vi "Add to Tree.vi"(8 "error in (no error)":errorcluster, 9 "Parent Tag":string, 10 "Tree Manager in":refnum<class "Tree Manager.lvclass">, 11 "Attribute in":refnum<class "Attribute.lvclass">) -> (0 "error out":errorcluster, 2 "Tree Manager out":refnum<class "Tree Manager.lvclass">, 3 "Attribute out":refnum<class "Attribute.lvclass">)   [LabVIEW 2023, in "VILab.lvlib" / "Attribute.lvclass"]
uses:
  Attribute.lvclass
  Tree Manager.lvclass
  Data Item.lvclass
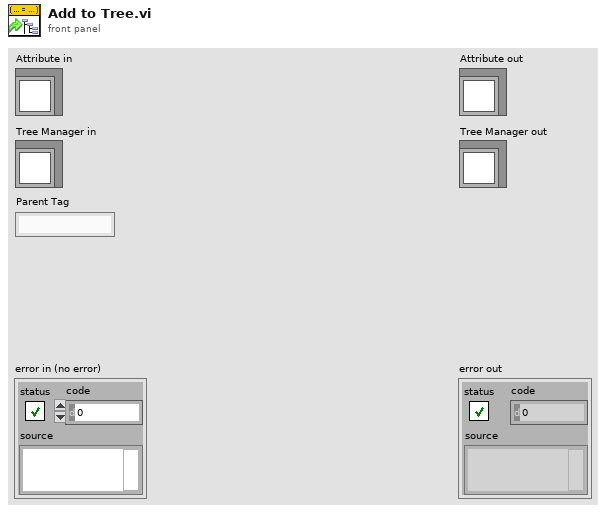
[diagram p1: front panel]
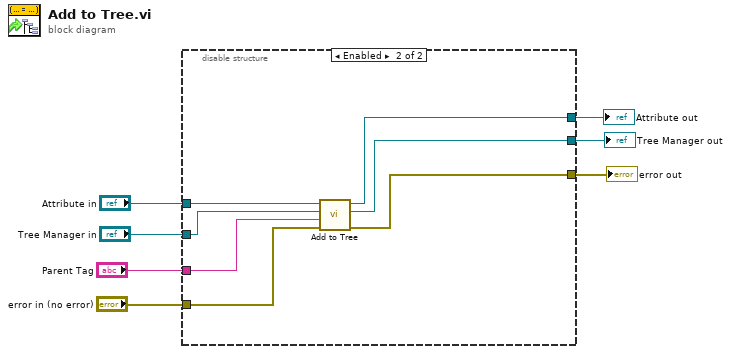
[diagram p0: block diagram]
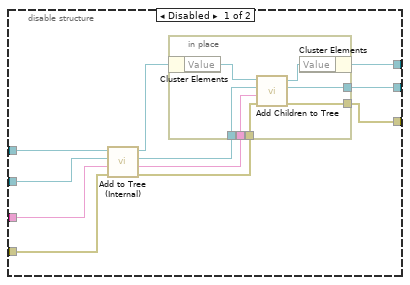
[diagram p2: hidden frame]
diagram:
  n1 = disable-structure shown="Enabled" {
    disable-tunnel: "Parent Tag" -> [w18 w30]
    disable-tunnel: "Tree Manager in" -> [w17 w31]
    disable-tunnel: "error in (no error)" -> [w16 w29]
    disable-tunnel: "Attribute in" -> [w15 w32]
    disable-tunnel: [w10 w28] -> w3
    disable-tunnel: [w9 w27] -> w2
    disable-tunnel: [w8 w26] -> w1
    frame Disabled {
      n2 = call "Add to Tree (Internal).vi"("error in (no error)"=w16, "Parent Tag"=w18, "Tree Manager in"=w17, "Data Item in"=w15) -> ("error out"=w13:errorcluster, "New Tag"=w11:string, "Tree Manager out"=w12:refnum<class "Tree Manager.lvclass">, "Data Item out"=w14:refnum<class "Attribute.lvclass">)  [unwired: 4 in]
      n3 = in-place {
        in-place-border: w13 -> [w23]
        in-place-border: w12 -> [w22]
        in-place-border: w11 -> [w21]
        in-place-border: [w20] -> w9
        in-place-border: [w19] -> w8
        n4 = in-place-cluster #1(w14) -> ("Value"=w25:refnum<class "Data Item.lvclass">)
        n5 = call "Add Children to Tree.vi"("error in (no error)"=w23, "Parent Tag"=w21, "Tree Manager in"=w22, "Data Item in"=w25) -> ("error out"=w19:errorcluster, "Tree Manager out"=w20:refnum<class "Tree Manager.lvclass">, "Data Item out"=w24:refnum<class "Data Item.lvclass">)  [unwired: 5 in]
        n6 = in-place-cluster #1("Value"=w24) -> (w10:refnum<class "Attribute.lvclass">)
      }
    }
    frame Enabled {
      n7 = call-parent "Add to Tree.vi"("error in (no error)"=w29, "Parent Tag"=w30, "Tree Manager in"=w31, "Data Item in"=w32) -> ("error out"=w26:errorcluster, "Tree Manager out"=w27:refnum<class "Tree Manager.lvclass">, "Data Item out"=w28:refnum<class "Attribute.lvclass">)  [unwired: 5 in]
    }
  }
  "error out" <- w1
  "Tree Manager out" <- w2
  "Attribute out" <- w3
